vi "stimulus.vi"(6 "error play 2":errorcluster, 7 "幅值(V)":dbl, 8 "stop frequency [Hz]":dbl, 9 "start frequency [Hz]":dbl, 10 "信号时长":dbl, 11 "Format":cluster{"Rate":i32, "Bits":i32, "Channels":u32}={"Rate"=44100, "Bits"=32, "Channels"=2}) -> (0 "error play 3":errorcluster caption="error play", 1 "stimulus":waveform(dbl) caption="输出波形", 2 "data length":i32, 3 "Output data":i32[][](array[numeric]))   [LabVIEW 2018]
uses:
  <vilib>/addons/_NISVFA/_Generation/SoundVib_Generation.lvlib
  <vilib>/Analysis/NI_AALPro.lvlib
  <vilib>/Analysis/4window.llb/Hamming Window (DBL).vi
panel:
  in  "信号时长(s)":dbl
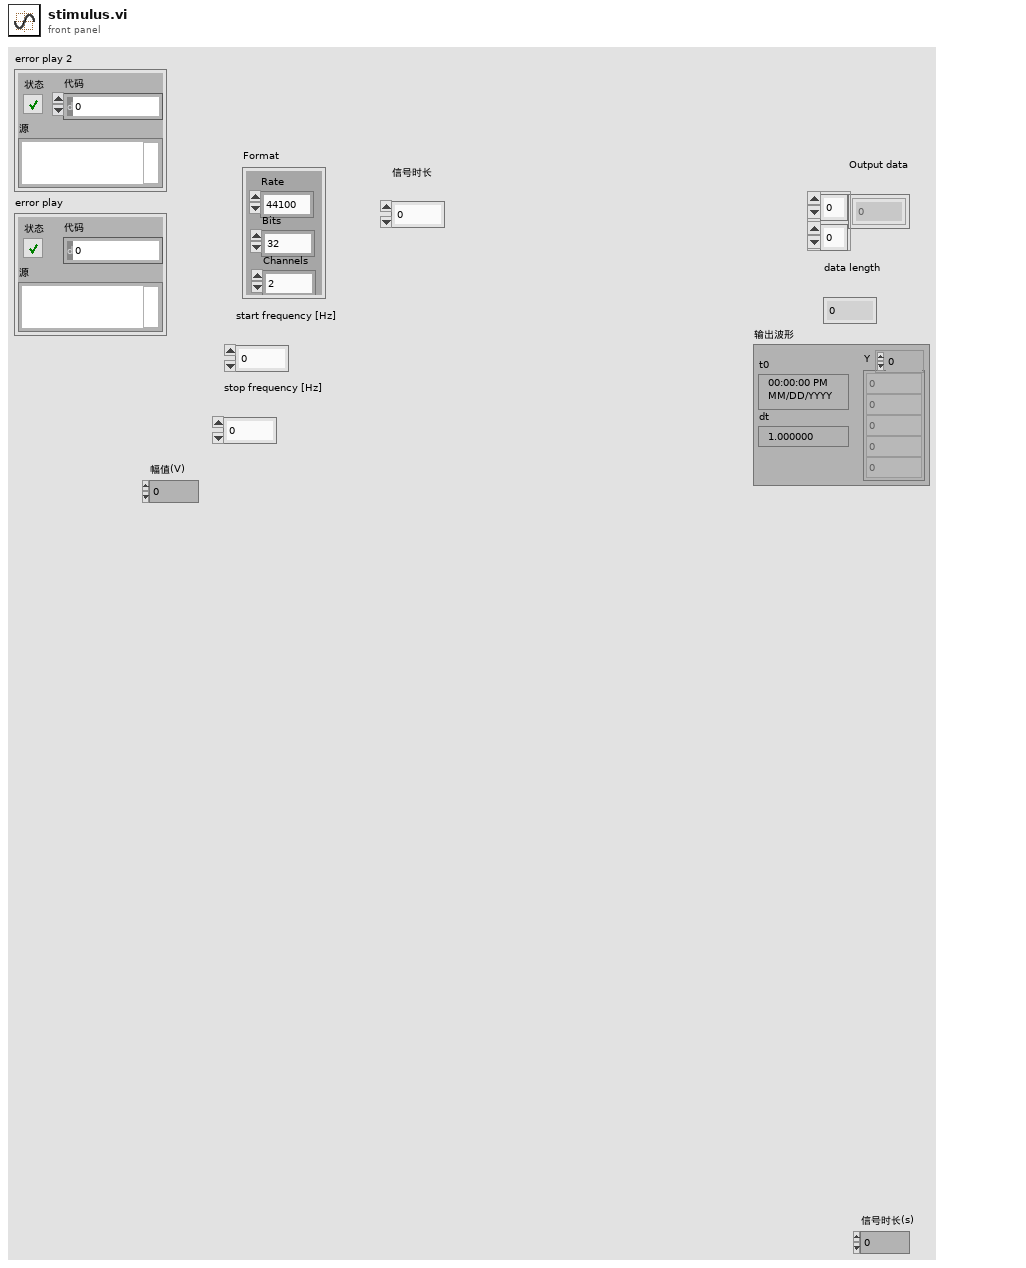
[diagram p1: front panel]
types:
  T1 = cluster{"start frequency [Hz]":dbl, "stop frequency [Hz]":dbl}
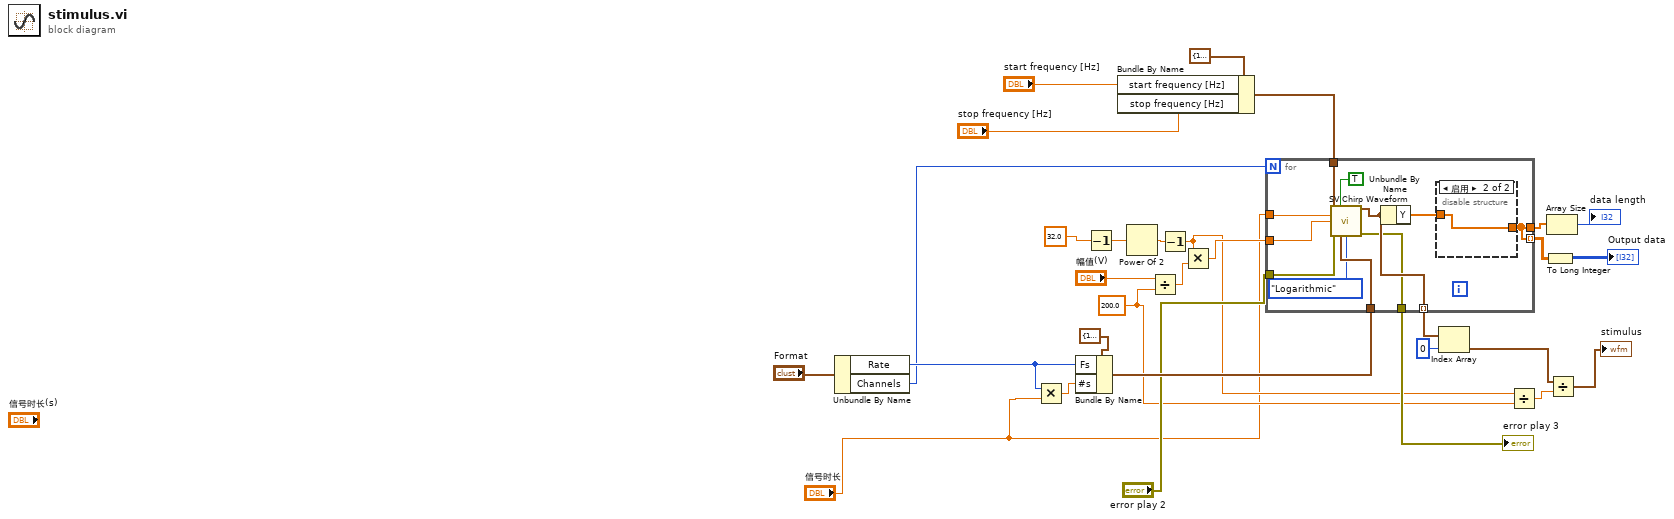
[diagram p0: block diagram]
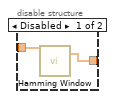
[diagram p2: hidden frame]
diagram:
  w7 = 200.0 ("y")
  n1 = Unbundle By Name("Format") -> ("Rate"=w22:i32, "Channels"=w18:u32)
  n2 = Multiply(x=w22, y="信号时长") -> (x*y=w25:dbl)
  n3 = Bundle By Name(cluster=cluster{"Fs":dbl, "#s":dbl} {"Fs"=1000.0, "#s"=1000.0} ("sampling info"), "Fs"=w22, "#s"=w25) -> (w21:cluster{"Fs":dbl, "#s":dbl})
  n4 = Decrement(x=32.0) -> (x-1=w27:dbl)
  n5 = Bundle By Name(cluster=T1 {"start frequency [Hz]"=10.0, "stop frequency [Hz]"=10000.0} ("frequency range"), "start frequency [Hz]"="start frequency [Hz]", "stop frequency [Hz]"="stop frequency [Hz]") -> (w19:T1)
  n6 = Power Of 2(x=w27) -> (2^x=w26:dbl)
  n7 = Divide(x="幅值(V)", y=w7) -> (x/y=w10:dbl)
  n8 = Decrement(x=w26) -> (x-1=w6:dbl)
  n9 = Multiply(x=w6, y=w10) -> (x*y=w28:dbl)
  n10 = for {
    N: w18 -> [_]
    tunnel: [w31] -> w4 mode=indexing
    tunnel: w28 -> [w40]
    tunnel: "信号时长" -> [w39]
    tunnel: [w31] -> w30
    tunnel: w21 -> [w38]
    tunnel: w19 -> [w36]
    tunnel: [w35] -> w16 mode=indexing
    tunnel: "error play 2" -> [w34]
    tunnel: [w33] -> w12
    n11 = call <vilib>:"SV Chirp Waveform.vi"("frequency range"=w36, "reset signal (F)"=TRUE ("reset signal"), "chirp duration [s]"=w39, "amplitude"=w40, "error in (no error)"=w34, "sampling info"=w38, "frequency spacing"=enum16{"Linear", "Logarithmic"}."Logarithmic") -> ("chirp signal"=w35:waveform(dbl), "error out"=w33:errorcluster)  [unwired: 6 in, 1 out]
    n12 = Unbundle By Name(w35) -> ("Y"=w32:dbl[])
    n13 = disable-structure shown="启用" {
      disable-tunnel: w32 -> [w43 w44]
      disable-tunnel: [w42 w44] -> w31
      frame Disabled {
        n14 = call-poly <vilib>:"Hamming Window.vi"("X"=w43) -> ("Windowed X"=w42:dbl[])  [unwired: 1 out]
      }
      frame Enabled {
      }
    }
  }
  "error play 3" <- w12
  n15 = Index Array(array=w16, index=0 ("索引")) -> (element=w9:waveform(dbl))
  n16 = Divide(x=w6, y=w7) -> (x/y=w8:dbl)
  n17 = To Long Integer(number=w4) -> (32bit integer=→"Output data":i32[][])
  n18 = Array Size(array=w30) -> (size(s)=→"data length":i32)
  n19 = Divide(x=w9, y=w8) -> (x/y=→"stimulus":waveform(dbl))
